vi "LakeShore_Test.vi"() -> ()   [LabVIEW 2009]
panel:
  out "Waveform Chart":dbl(graph)
  out "Temperature [C]":dbl
  in  "End Program":bool
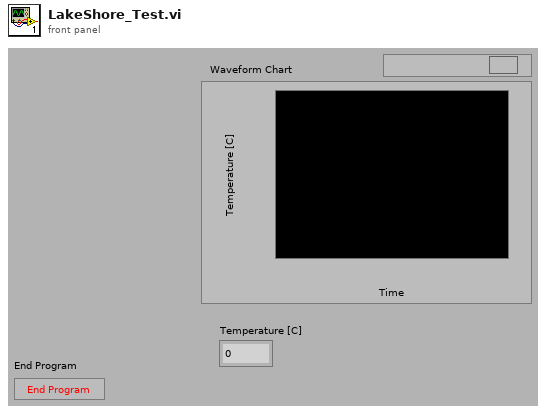
[diagram p1: front panel]
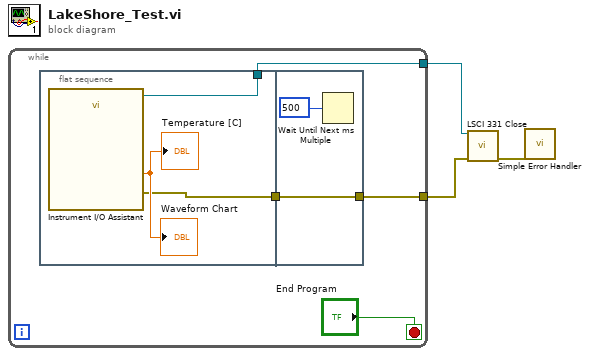
[diagram p0: block diagram]
diagram:
  n1 = while {
    tunnel: [w7] -> w3
    tunnel: [w6] -> w2
    stop <- "End Program" stop-if-true
    n2 = flat-sequence {
      tunnel: [w9] -> w7
      tunnel: [w8] -> w5
      tunnel: [w11] -> w6
      tunnel: w5 -> [w11]
      frame #0 {
        n3 = call "Instrument I/O Assistant"() -> ("Session Out"=w9:refnum<visa-resource-name>, "Temperature [C]"=→"Temperature [C]" →"Waveform Chart":dbl, "error out"=w8:errorcluster)  [unwired: 25 in]
      }
      frame #1 {
        n4 = Wait Until Next ms Multiple(millisecond multiple=u32 500) -> ()  [unwired: 1 out]
      }
    }
  }
  n5 = call "LSCI 331 Close.vi"("VISA session"=w3, "error in (no error)"=w2) -> ("error out"=w1:errorcluster)  [unwired: 13 in]
  n6 = call <vilib>:"Simple Error Handler.vi"("error in (no error)"=w1) -> ()  [unwired: 4 in, 5 out]
